vi "Autodetect.vi"(8 "error in":errorcluster) -> (0 "error out":errorcluster, 3 "IP Addresses":string[](array[string]))   [LabVIEW 2014, in "Raspberry Pi Compatible Compiler for LabVIEW.lvlib" / "Autodetect.lvlib"]
doc: "Launches the home page for each detected device"
uses:
  Autodetect.lvlib
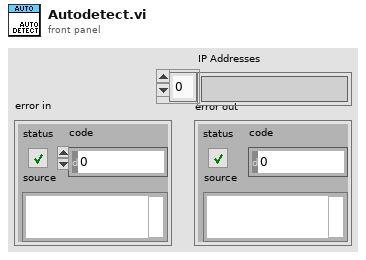
[diagram p1: front panel]
types:
  T1 = typedef "Raspberry Pi Compatible Compiler for LabVIEW.lvlib/Autodetect.lvlib/UDP_Response_TD.ctl" = cluster{"IP address":string, "Port":u16, "response":string}
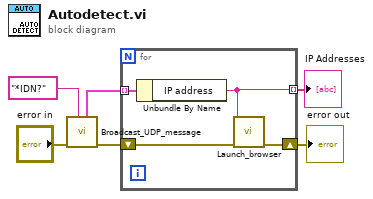
[diagram p0: block diagram]
diagram:
  n1 = call "Broadcast_UDP_message.vi"("message"="*IDN?", "error in"="error in") -> ("error out"=w5:errorcluster, "responses"=w6:T1[])  [unwired: 6 in]
  n2 = for {
    tunnel: w6 -> [w10] mode=indexing
    shift-right: [w8] -> w3
    shift-left: w5 -> [w9]
    tunnel: [w7] -> w1 mode=indexing
    n3 = Unbundle By Name(w10) -> ("IP address"=w7:string)
    n4 = call "Launch_browser.vi"("error in"=w9, "host address"=w7) -> ("error out"=w8:errorcluster)  [unwired: 6 in, 1 out]
  }
  "error out" <- w3
  "IP Addresses" <- w1
